vi "Frame Read.vi"(8 "error in (no error)":errorcluster caption="entrée d'erreur (pas d'erreur)", 10 "Frame Read":string, 11 "Class Camera  IV3-500CA - Start Program en Entrée":refnum<class "Class Camera  IV3-500CA - Start Program.lvclass">) -> (0 "error out":errorcluster caption="sortie d'erreur", 3 "Class Camera  IV3-500CA - Start Program en Sortie":refnum<class "Class Camera  IV3-500CA - Start Program.lvclass">)   [LabVIEW 2020, in "Library Instrument & Equipement.lvlib" / "Library Camera.lvlib" / "Class Camera  IV3-500CA - Start Program.lvclass"]
uses:
  Class Camera  IV3-500CA - Start Program.lvclass
  Class Camera  IV3-500CA - Start Program.lvclass/Class Camera  IV3-500CA - Start Program.ctl
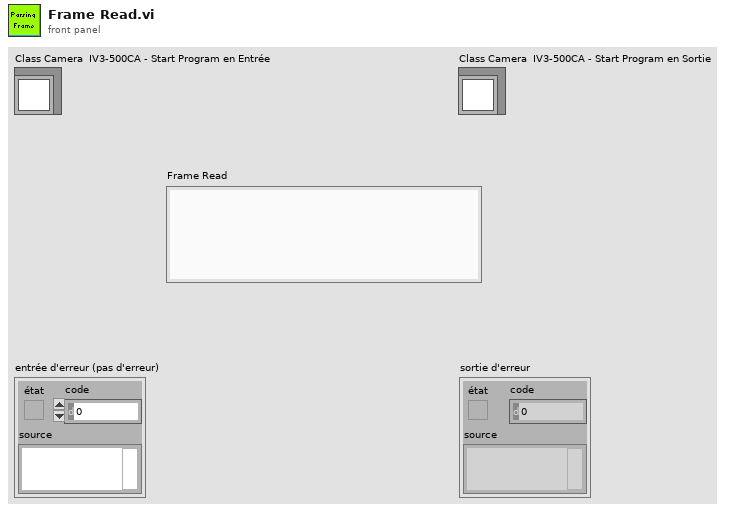
[diagram p1: front panel]
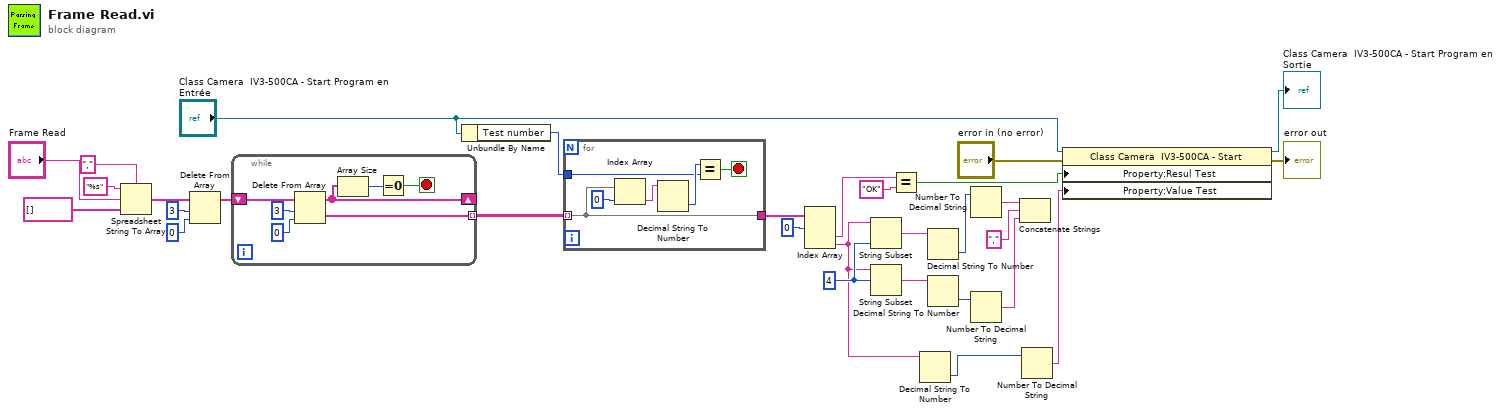
[diagram p0: block diagram]
diagram:
  w16 = 4 ("longueur (reste)")
  n1 = Spreadsheet String To Array(delimiter (Tab)="," ("séparateur (Tabulation)"), format string="%s" ("chaîne de format"), spreadsheet string="Frame Read", array type (2D Dbl)=string[] []) -> (array=w27:string[])
  n2 = Delete From Array(array=w27, length=3 ("longueur"), index=0 ("indice")) -> (array with subset deleted=w24:string[])  [unwired: 1 out]
  n3 = while {
    shift-right: [w34] -> _
    shift-left: w24 -> [w37]
    tunnel: [w31] -> w9 mode=indexing
    stop <- w32 stop-if-true
    n4 = Delete From Array(array=w37, length=3 ("longueur"), index=0 ("indice")) -> (deleted portion=w31:string[], array with subset deleted=w34:string[])
    n5 = Array Size(array=w34) -> (size(s)=w33:i32)
    n6 = Equal To 0?(x=w33) -> (x = 0?=w32:bool)
  }
  n7 = Unbundle By Name("Class Camera  IV3-500CA - Start Program en Entrée") -> ("Test number"=w4:u16)
  n8 = for {
    tunnel: w9 -> [w38] mode=indexing
    tunnel: w4 -> [w40]
    tunnel: [w38] -> w8
    stop <- w39 stop-if-true
    n9 = Index Array(array=w38, index=0 ("indice")) -> (element=w42:string)
    n10 = Decimal String To Number(string=w42) -> (number=w41:i32)  [unwired: 2 in, 1 out]
    n11 = Equal?(x=w41, y=w40) -> (x = y?=w39:bool)
  }
  n12 = Index Array(array=w8, index #1=0 ("indice")) -> (element #2=w21:string, element #3=w3:string)  [unwired: 2 in, 1 out]
  n13 = String Subset(string=w3, length (rest)=w16) -> (substring=w17:string)  [unwired: 1 in]
  n14 = String Subset(string=w3, offset (0)=w16) -> (substring=w15:string)  [unwired: 1 in]
  n15 = Equal?(x=w21, y="OK") -> (x = y?=w18:bool)
  n16 = Decimal String To Number(string=w3) -> (number=w2:i32)  [unwired: 2 in, 1 out]
  n17 = Decimal String To Number(string=w17) -> (number=w14:i32)  [unwired: 2 in, 1 out]
  n18 = Decimal String To Number(string=w15) -> (number=w10:i32)  [unwired: 2 in, 1 out]
  n19 = Number To Decimal String(number=w14) -> (decimal integer string=w13:string)  [unwired: 1 in]
  n20 = Number To Decimal String(number=w10) -> (decimal integer string=w11:string)  [unwired: 1 in]
  n21 = Concatenate Strings(w13, "," ("chaîne"), w11) -> ()  [unwired: 1 out]
  n22 = Number To Decimal String(number=w2) -> (decimal integer string=w1:string)  [unwired: 1 in]
  n23 = property class="Class Camera  IV3-500CA - Start"(reference="Class Camera  IV3-500CA - Start Program en Entrée", error in="error in (no error)", "Property:Resul Test "=w18, "Property:Value Test"=w1) -> (reference out=→"Class Camera  IV3-500CA - Start Program en Sortie":refnum<class "Class Camera  IV3-500CA - Start Program.lvclass">, error out=→"error out":errorcluster)
